vi "URAPI_IfThen.vi"(0 "Variable In":string="voltage", 1 "Compare to":string="voltage", 3 "URAPI Script":T1={"Script"="", "Whiles"=[], "Ifs"=[], "Supress Err"=TRUE, "Errors"=""}, 4 "Comparison":enum16{">", "<", ">=", "<=", "=", "!="}(ring)) -> (2 "URAPI False":T1={"Script"="", "Whiles"=[], "Ifs"=[], "Supress Err"=TRUE, "Errors"=""}, 5 "URAPI True":T1={"Script"="", "Whiles"=[], "Ifs"=[], "Supress Err"=TRUE, "Errors"=""})   [LabVIEW 2012]
doc: "Compares \"Variable in\" to \"Compare to\" with specified \"Comparison\" constant. If true, script follows \"URAPI True\" path, and \"URAPI False\" if false."
uses:
  <userlib>/BotSpeak/VIs/Direct/URAPI_Control.ctl
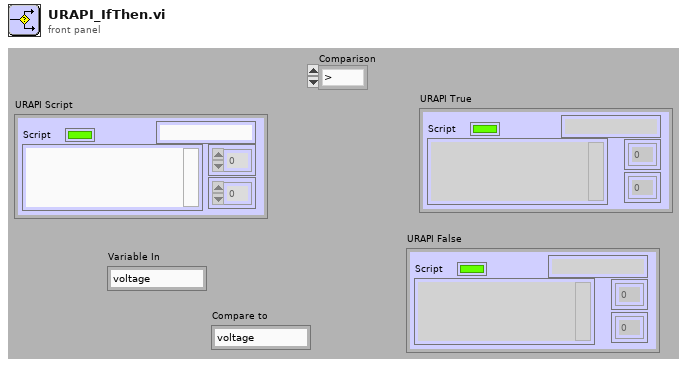
[diagram p1: front panel]
types:
  T1 = typedef "URAPI_Control.ctl" = cluster{"Script":string, "Whiles":u8[], "Ifs":u8[], "Supress Err":bool, "Errors":string}
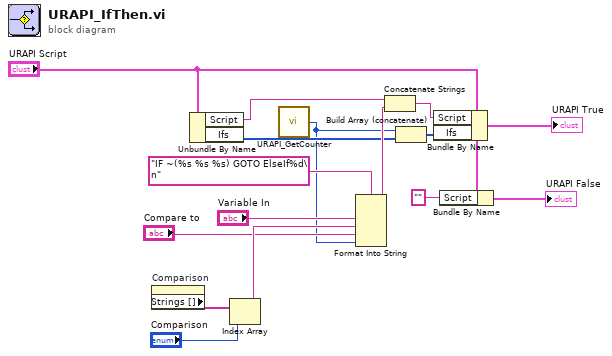
[diagram p0: block diagram]
diagram:
  n1 = property on="Comparison" class="Enum (strict)"() -> ("Strings []"=w9:string[])  [unwired: 2 in, 2 out]
  n2 = Unbundle By Name("URAPI Script") -> ("Script"=w4:string, "Ifs"=w3:u8[])
  n3 = Index Array(array=w9, index="Comparison") -> (element=w7:string)
  n4 = call <userlib>:"URAPI_GetCounter.vi"() -> ("Numeric"=w1:u16)  [unwired: 1 in]
  n5 = Format Into String(format string="IF ~(%s %s %s) GOTO ElseIf%d\n" ("string"), "Variable In", w7, "Compare to", w1) -> (resulting string=w5:string)  [unwired: 2 in, 1 out]
  n6 = Concatenate Strings(w4, w5) -> (w13:string)
  n7 = Build Array (concatenate)(w1, w3) -> (w2:u16[])
  n8 = Bundle By Name(cluster="URAPI Script", "Script"=w13, "Ifs"=w2) -> (→"URAPI True":T1)
  n9 = Bundle By Name(cluster="URAPI Script", "Script"="" ("string")) -> (→"URAPI False":T1)
